vi "Write daemon status.vi"(8 "error in (no error)":errorcluster, 10 "daemon status":T1(ring), 11 "network slave in":refnum<class "Network Slave.lvclass">) -> (0 "error out":errorcluster, 3 "network slave out":refnum<class "Network Slave.lvclass">)   [LabVIEW 2020, in "SubVIs.lvlib" / "Network Slave.lvclass"]
uses:
  <vilib>/Modbus/subvis/Protocol/Interfaces/Network Slave/Network Slave.lvclass
  <vilib>/Modbus/subvis/Protocol/Interfaces/Network Slave/Network Slave.lvclass/Network Slave.ctl
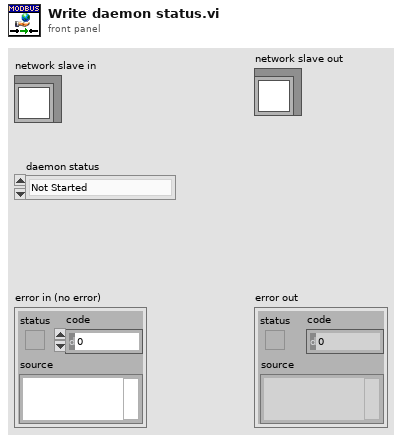
[diagram p1: front panel]
types:
  T1 = enum16{"Not Started", "Running", "Error", "Stopped"}
  T2 = typedef "SubVIs.lvlib/Network Slave.lvclass/daemon status cluster.ctl" = cluster{"error":errorcluster, "status":enum16{"Not Started", "Running", "Error", "Stopped"}}
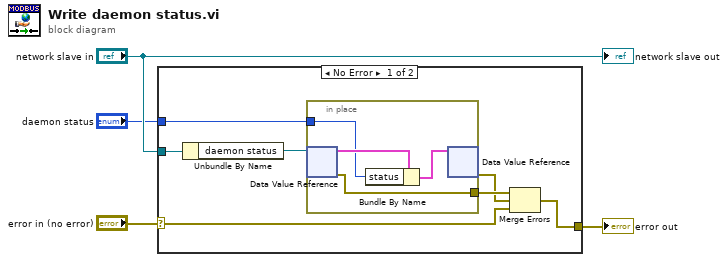
[diagram p0: block diagram]
diagram:
  n1 = case shown="No Error" "error in (no error)" {
    selector: "error in (no error)" -> [w6 w16]
    tunnel: [w10 w16] -> w4
    tunnel: "network slave in" -> [w9 _]
    tunnel: "daemon status" -> [w8 _]
    frame No Error {
      n2 = Unbundle By Name(w9) -> ("daemon status"=w11:refnum<data-value>)
      n3 = in-place {
        in-place-border: w8 -> [w13]
        in-place-border: [w12] -> w7
        n4 = in-place-dvr #1(w11) -> (w15:T2, w12:errorcluster)
        n5 = Bundle By Name(cluster=w15, "status"=w13) -> (w14:T2)
        n6 = in-place-dvr #1(w14) -> (w5:errorcluster)  [unwired: 1 out]
      }
      n7 = Merge Errors(w7, w5, w6) -> (w10:errorcluster)
    }
    frame Error {
    }
  }
  "error out" <- w4
  "network slave out" <- "network slave in"
